vi "Update.vi"(8 "error in (no error)":errorcluster, 9 "Reobserved Array":bool[](array[boolean]), 10 "SLAM In":T1, 11 "Y":T2) -> (0 "error out":errorcluster, 2 "SLAM Out":T1)   [LabVIEW 2009]
uses:
  Controls/SLAM.ctl
  <vilib>/Analysis/Matrix/Datatypes/RealMatrix.ctl
  <vilib>/Analysis/Matrix/Numeric/Add/Add - RM,RM.vi
  <vilib>/Analysis/baseanly.llb/Real A x B.vi
  <vilib>/Analysis/Matrix/Numeric/Subtract/Subtract - RM,RM.vi
  <vilib>/Analysis/NI_AALBase.lvlib
  <vilib>/Analysis/Matrix/NI_Matrix.lvlib
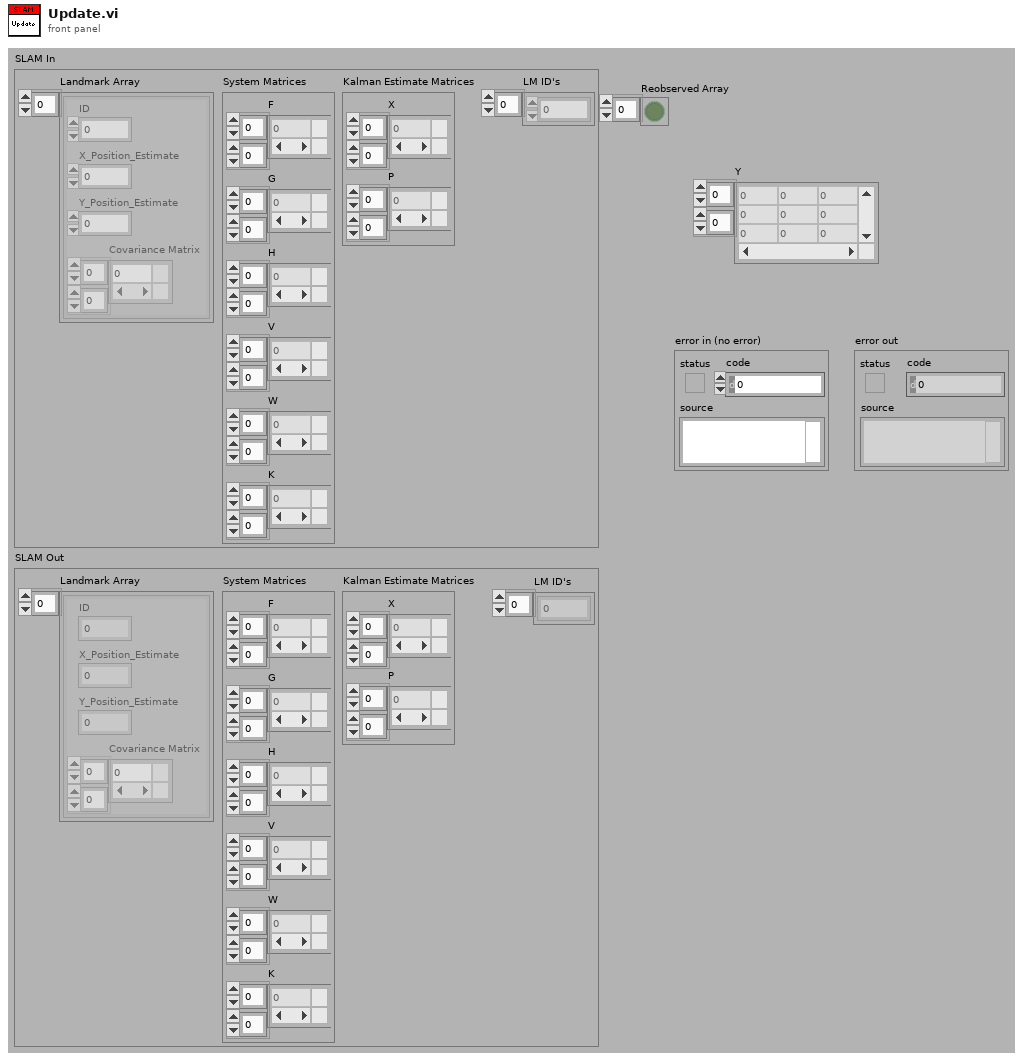
[diagram p1: front panel]
types:
  T1 = typedef "SLAM.ctl" = cluster{"Landmark Array":cluster{"ID":dbl, "X_Position_Estimate":dbl, "Y_Position_Estimate":dbl, "Covariance Matrix":T2}[], "System Matrices":cluster{"F":T2, "G":T2, "H":T2, "V":T2, "W":T2, "K":T2}, "Kalman Estimate Matrices":cluster{"X":T2, "P":T2}, "LM ID's":dbl[]}
  T2 = typedef "NI_Matrix.lvlib/RealMatrix.ctl" = dbl[][]
  T3 = cluster{"F":T2, "G":T2, "H":T2, "V":T2, "W":T2, "K":T2}
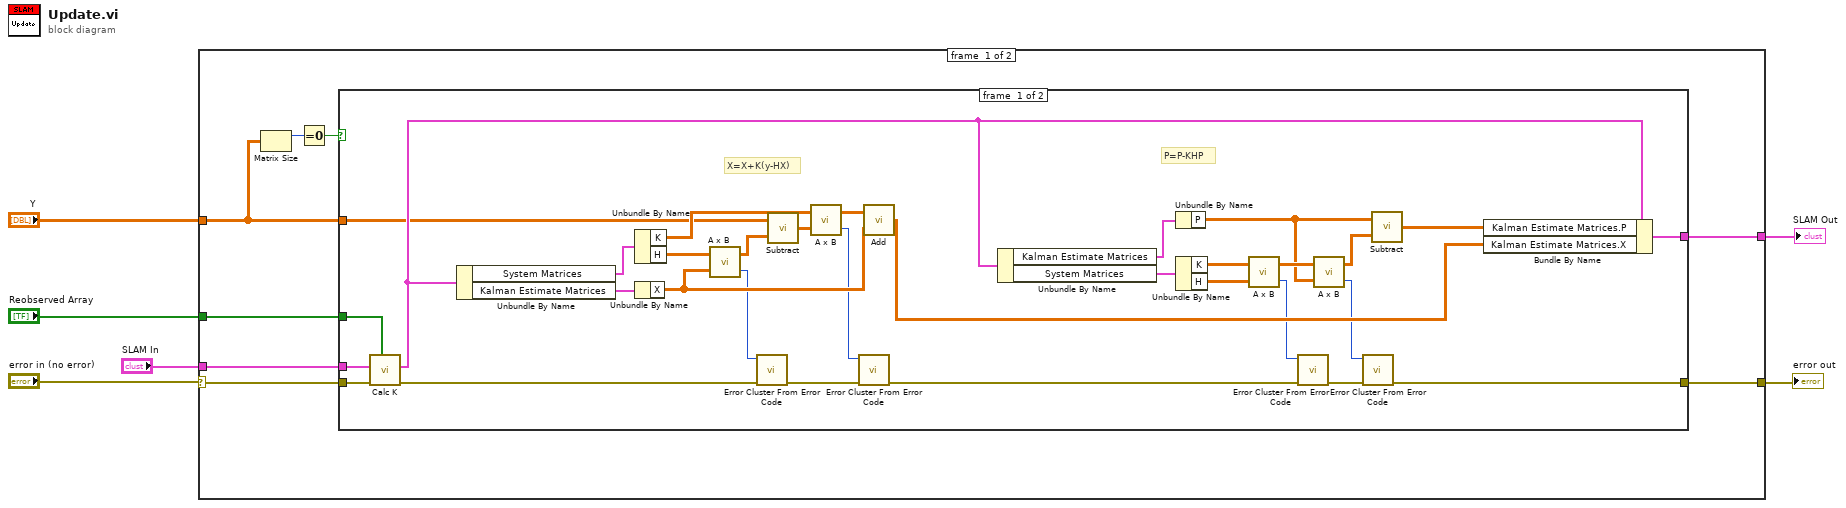
[diagram p0: block diagram]
diagram:
  n1 = case shown="No Error" "error in (no error)" {
    selector: "error in (no error)" -> [w14 w50]
    tunnel: [w13 w50] -> w5
    tunnel: "SLAM In" -> [w12 w49]
    tunnel: [w11 w49] -> w3
    tunnel: "Reobserved Array" -> [w10 _]
    tunnel: "Y" -> [w9 _]
    frame #0 {
      n2 = Matrix Size(0:w9) -> (1:w8:i32)  [unwired: 1 out]
      n3 = Equal To 0?(x=w8) -> (x = 0?=w7:bool)
      n4 = case shown="True" w7 {
        tunnel: w14 -> [w44 w48]
        tunnel: [w19 w48] -> w13
        tunnel: w12 -> [w18 w47]
        tunnel: [w17 w47] -> w11
        tunnel: w10 -> [w16 _]
        tunnel: w9 -> [w15 _]
        frame #0 {
          # "P=P-KHP"
          # "X=X+K(y-HX)"
          n5 = call "Calc K.vi"("Reobserved Array"=w16, "error in (no error)"=w44, "SLAM In"=w18) -> ("error out"=w36:errorcluster, "SLAM Out"=w32:T1)  [unwired: 7 in]
          n6 = Unbundle By Name(w32) -> ("System Matrices"=w45:T3, "Kalman Estimate Matrices"=w46:cluster{"X":T2, "P":T2})
          n7 = Unbundle By Name(w45) -> ("K"=w40:T2, "H"=w43:T2)
          n8 = Unbundle By Name(w46) -> ("X"=w38:T2)
          n9 = call-poly <vilib>:"A x B.vi"("B"=w38, "A"=w43) -> ("error"=w35:i32, "A x B"=w42:T2)
          n10 = call <vilib>:"Error Cluster From Error Code.vi"("error in (no error)"=w36, "error code (0)"=w35) -> ("error out"=w33:errorcluster)  [unwired: 7 in]
          n11 = call-poly <vilib>:"Subtract.vi"("Real Matrix B"=w42, "Real Matrix A"=w15) -> ("A - B"=w41:T2)
          n12 = call-poly <vilib>:"A x B.vi"("B"=w41, "A"=w40) -> ("error"=w34:i32, "A x B"=w39:T2)
          n13 = call <vilib>:"Error Cluster From Error Code.vi"("error in (no error)"=w33, "error code (0)"=w34) -> ("error out"=w21:errorcluster)  [unwired: 7 in]
          n14 = call-poly <vilib>:"Add.vi"("Real Matrix B"=w38, "Real Matrix A"=w39) -> ("A + B"=w24:T2)
          n15 = Unbundle By Name(w32) -> ("Kalman Estimate Matrices"=w31:cluster{"X":T2, "P":T2}, "System Matrices"=w37:T3)
          n16 = Unbundle By Name(w31) -> ("P"=w27:T2)
          n17 = Unbundle By Name(w37) -> ("K"=w30:T2, "H"=w29:T2)
          n18 = call-poly <vilib>:"A x B.vi"("B"=w29, "A"=w30) -> ("error"=w23:i32, "A x B"=w28:T2)
          n19 = call <vilib>:"Error Cluster From Error Code.vi"("error in (no error)"=w21, "error code (0)"=w23) -> ("error out"=w20:errorcluster)  [unwired: 7 in]
          n20 = call-poly <vilib>:"A x B.vi"("B"=w27, "A"=w28) -> ("error"=w22:i32, "A x B"=w26:T2)
          n21 = call <vilib>:"Error Cluster From Error Code.vi"("error in (no error)"=w20, "error code (0)"=w22) -> ("error out"=w19:errorcluster)  [unwired: 7 in]
          n22 = call-poly <vilib>:"Subtract.vi"("Real Matrix B"=w26, "Real Matrix A"=w27) -> ("A - B"=w25:T2)
          n23 = Bundle By Name(cluster=w32, "Kalman Estimate Matrices.P"=w25, "Kalman Estimate Matrices.X"=w24) -> (w17:T1)
        }
        frame #1 {
        }
      }
    }
    frame #1 {
    }
  }
  "error out" <- w5
  "SLAM Out" <- w3
